vi "Command - Continuous (SubVI) - A.vi"(0 "ESP Config":T1={"COM Port Input"="COM8", "Manual Command"={"Device Type"="", "Instance"="", "Command"="", "Sub-Command"="", "Parameters (Seperate by :)"=""}, "Device Type"="e", "Instance"="a", "Use Manual Command"=FALSE, "Timeout [msec]"=1000, "Read/Write Wait [msec]"=50}, 5 "ESP Table Cluster Ref":refnum<vi>, 7 "Display Cluster Ref":refnum<vi>) -> (4 "ESP Values":T2, 6 "Parameters":string[][](array[string]), 8 "Continuous Header":string[](array[string]), 10 "Continuous Data":string[](array[string]), 15 "CONTINUOUS ERR":errorcluster)   [LabVIEW 2011]
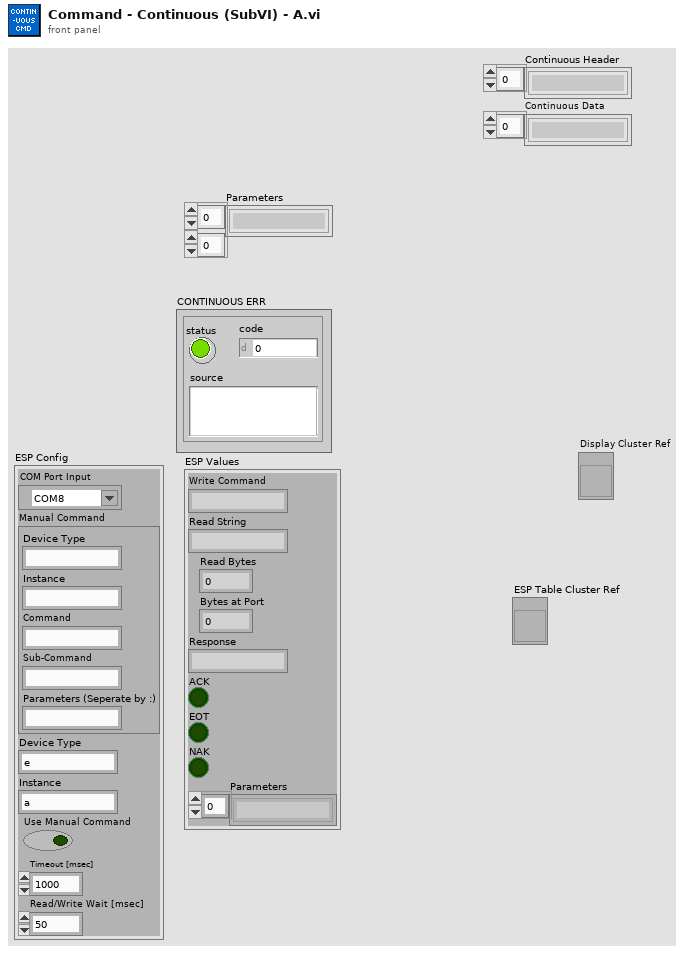
[diagram p1: front panel]
types:
  T1 = cluster{"COM Port Input":refnum<visa-resource-name>, "Manual Command":cluster{"Device Type":string, "Instance":string, "Command":string, "Sub-Command":string, "Parameters (Seperate by :)":string}, "Device Type":string, "Instance":string, "Use Manual Command":bool, "Timeout [msec]":u32, "Read/Write Wait [msec]":u32}
  T2 = cluster{"Write Command":string, "Read String":string, "Read Bytes":u32, "Bytes at Port":u32, "Response":string, "ACK":bool, "EOT":bool, "NAK":bool, "Parameters":string[]}
  T3 = cluster{"ON Demand Button":i32, "ON Demand Commands":i32, "Continuous Button":i32, "Continuous Commands":i32, "Error Button":i32, "Error Command":i32, "Status Button":i32, "Status Command":i32, "Digital Button":i32, "Digital Command":i32, "Save Table Button":i32, "Active Table":i32, "New Table Name":i32, "Table":i32}
  T4 = cluster{"Device Type":string, "Instance":string, "Command":string, "Sub-Command":string, "Parameters (Seperate by :)":string}
  T5 = cluster{"CMD_Display":string, "Param Output":string[][]}[]
  T6 = cluster{"ParamName":string, "Param Output":string[][]}
  T7 = cluster{"ParamName":string, "Param Output":string[][]}[]
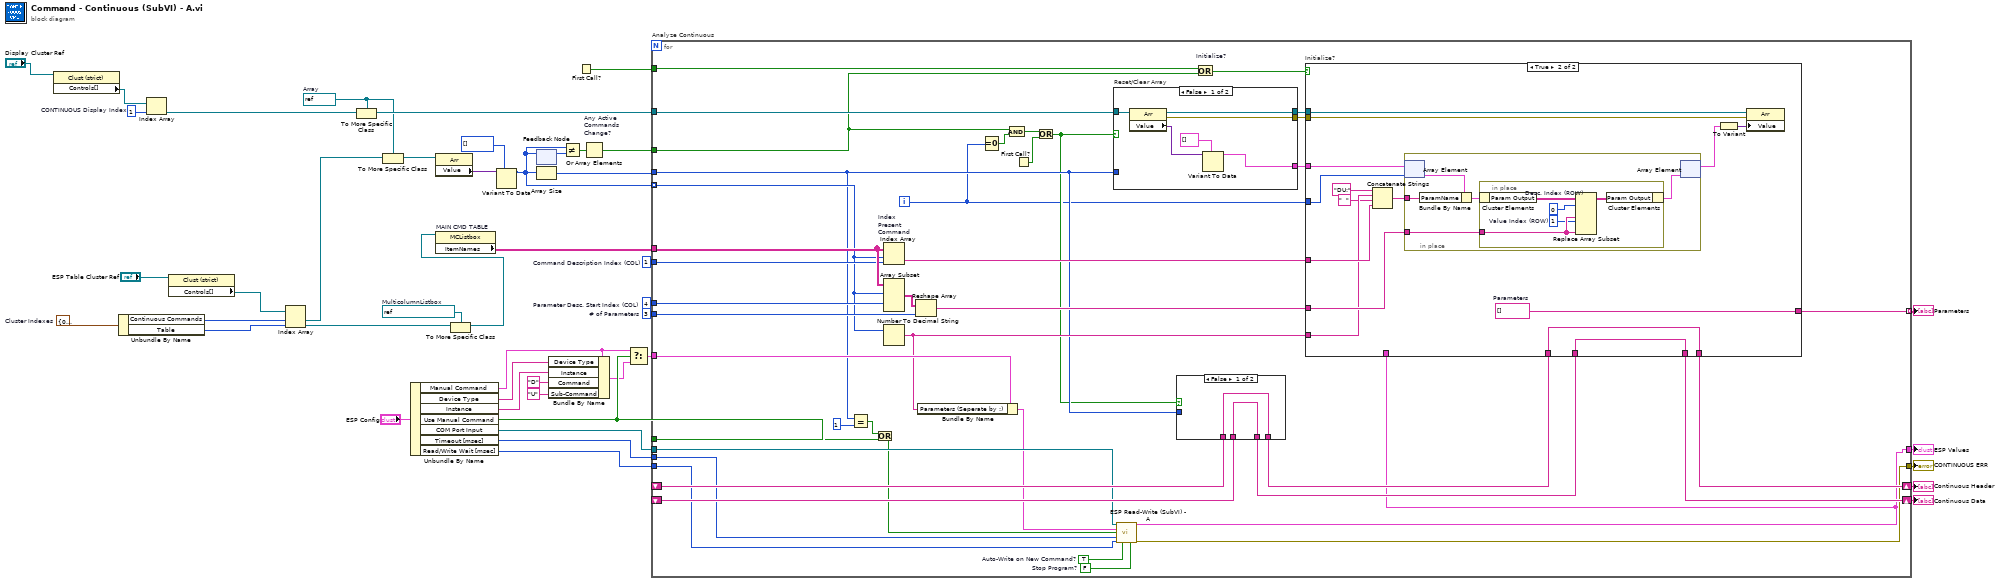
[diagram p0: block diagram]
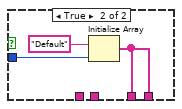
[diagram p2: hidden frame]
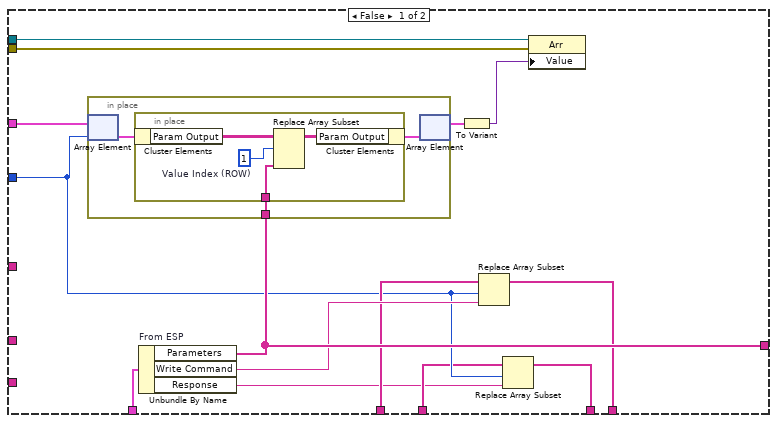
[diagram p3: hidden frame]
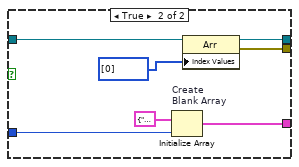
[diagram p4: hidden frame]
diagram:
  w9 = 1  # CONTINUOUS Display Index
  w12 = refnum<vi> refnum  # MulticolumnListbox
  w17 = T3 {"ON Demand Button"=0, "ON Demand Commands"=1, "Continuous Button"=2, "Continuous Commands"=3, "Error Button"=4, "Error Command"=5, "Status Button"=6, "Status Command"=7, "Digital Button"=8, "Digital Command"=9, "Save Table Button"=10, "Active Table"=11, "New Table Name"=12, "Table"=13}  # Cluster Indexes
  w4 = refnum<vi> refnum  # Array
  w43 = 1  # Command Description Index (COL)
  w44 = 3  # # of Parameters
  w45 = 4  # Parameter Desc. Start Index (COL)
  n1 = property class="Clust (strict)"(reference="Display Cluster Ref") -> ("Controls[]"=w10:refnum<vi>[])  [unwired: 1 in, 2 out]
  n2 = Unbundle By Name(w17) -> ("Continuous Commands"=w16:i32, "Table"=w15:i32)
  n3 = Index Array(array=w10, index=w9) -> (element=w8:refnum<vi>)
  n4 = property class="Clust (strict)"(reference="ESP Table Cluster Ref") -> ("Controls[]"=w18:refnum<vi>[])  [unwired: 1 in, 2 out]
  n5 = Index Array(array=w18, index #1=w16, index #2=w15) -> (element #1=w2:refnum<vi>, element #2=w13:refnum<vi>)
  n6 = To More Specific Class(target class=w4, reference=w8) -> (specific class reference=w19:refnum<vi>)  [unwired: 1 in, 1 out]
  n7 = To More Specific Class(target class=w4, reference=w2) -> (specific class reference=w5:refnum<vi>)  [unwired: 1 in, 1 out]
  n8 = Unbundle By Name("ESP Config") -> ("Manual Command"=w32:T4, "Device Type"=w34:string, "Instance"=w33:string, "Use Manual Command"=w39:bool, "COM Port Input"=w40:refnum<visa-resource-name>, "Timeout [msec]"=w41:u32, "Read/Write Wait [msec]"=w42:u32)
  n9 = property class="Arr"(reference=w5) -> ("Value"=w6:variant)  [unwired: 1 in, 2 out]
  n10 = To More Specific Class(target class=w12, reference=w13) -> (specific class reference=w11:refnum<vi>)  [unwired: 1 in, 1 out]
  n11 = property on="MAIN CMD TABLE" class="MCListbox"(reference=w11) -> ("ItemNames"=w25:string[][])  [unwired: 1 in, 2 out]
  n12 = Variant To Data(type=i32[] [], Variant=w6) -> (data=w3:i32[])  [unwired: 1 in, 1 out]
  n13 = feedback #1() -> (w27:i32[])  [unwired: 1 in]
  n14 = feedback-in #1(w3) -> ()
  n15 = Array Size(array=w3) -> (size(s)=w28:i32)
  n16 = Bundle By Name(cluster=w32, "Device Type"=w34, "Instance"=w33, "Command"="D", "Sub-Command"="U") -> (w31:T4)
  n17 = Not Equal?(x=w3, y=w27) -> (x != y?=w26:bool[])
  n18 = First Call?() -> (First Call?: T/F=w30:bool)
  n19 = Or Array Elements "Any Active\nCommands\nChange?"(Boolean array=w26) -> (logical OR=w29:bool)
  n20 = Select(t=w32, s=w39, f=w31) -> (s? t:f=w37:T4)
  n21 = for "Analyze Continuous" {
    tunnel: w25 -> [w86]
    tunnel: w30 -> [w80]
    tunnel: w19 -> [w79]
    tunnel: w28 -> [w64]
    tunnel: w45 -> [w83]
    tunnel: w37 -> [w87]
    tunnel: [w47] -> w23
    tunnel: w41 -> [w52]
    tunnel: w44 -> [w82]
    tunnel: w29 -> [w74]
    tunnel: w39 -> [w53]
    tunnel: w40 -> [w55]
    tunnel: w42 -> [w51]
    tunnel: w3 -> [w67] mode=indexing
    tunnel: w43 -> [w68]
    tunnel: [w65] -> w22 mode=indexing
    tunnel: [w48] -> w24
    shift-right: [w56] -> w21
    shift-left: _ -> [w62]
    shift-right: [w57] -> w20
    shift-left: _ -> [w61]
    i -> [w60]
    w49 = FALSE  # Stop Program?
    w50 = TRUE  # Auto-Write on New Command?
    n22 = Equal?(x=w64, y=1) -> (x = y?=w72:bool)
    n23 = Or(x=w72, y=w53) -> (x .or. y?=w46:bool)
    n24 = Index Array "Index\nPresent\nCommand"(array=w86, index (row)=w67, index (col)=w68) -> (element=w66:string)
    n25 = Array Subset(array=w86, index (row)=w67, index (col)=w83) -> (w85:string[][])  [unwired: 2 in]
    n26 = Number To Decimal String(number=w67) -> (decimal integer string=w81:string)  [unwired: 1 in]
    n27 = Reshape Array(w85, w82) -> (w84:string[])
    n28 = Bundle By Name(cluster=w87, "Parameters (Seperate by :)"=w81) -> (w54:T4)
    n29 = Equal To 0?(x=w60) -> (x = 0?=w78:bool)
    n30 = And(x=w74, y=w78) -> (x .and. y?=w71:bool)
    n31 = First Call?() -> (First Call?: T/F=w70:bool)
    n32 = Or(x=w71, y=w70) -> (x .or. y?=w63:bool)
    n33 = case "Reset/Clear Array" shown="False" w63 {
      tunnel: w79 -> [w144 w149]
      tunnel: [w143 w147] -> w75
      tunnel: [w142 w148] -> w76
      tunnel: [w139 w150] -> w77
      tunnel: w64 -> [_ w151]
      frame False {
        n34 = property class="Arr"(reference=w144) -> (reference out=w142:refnum<vi>, error out=w143:errorcluster, "Value"=w141:variant)  [unwired: 1 in]
        n35 = Variant To Data(type=T5 [], Variant=w141) -> (data=w139:T5)  [unwired: 1 in, 1 out]
      }
      frame True {
        n36 = Initialize Array "Create\nBlank Array"(T6 {"ParamName"="", "Param Output"=[["", "", ""], [" ", "", ""]]} ("Read Value\nCluster"), w151) -> (w150:T7)
        n37 = property class="Arr"(reference=w149, "Index Values"=u32[] [0]) -> (reference out=w148:refnum<vi>, error out=w147:errorcluster)  [unwired: 1 in]
      }
    }
    n38 = call "ESP Read-Write (SubVI) - A.vi"("COM Port Input"=w55, "Command Input"=w54, "Manual Write Command"=w46, "Timeout (ms)"=w52, "Write/Read Wait (ms)"=w51, "Auto-Write on New Command?"=w50, "Stop Program?"=w49) -> ("ESP Values"=w47:T2, "Error Output"=w48:errorcluster)  [unwired: 7 in]
    n39 = case shown="False" w63 {
      tunnel: w64 -> [_ w92]
      tunnel: [w88 w90] -> w58
      tunnel: [w89 w90] -> w59
      tunnel: w62 -> [w89 _]
      tunnel: w61 -> [w88 _]
      frame False {
      }
      frame True {
        n40 = Initialize Array("Default", w92) -> (w90:string[])
      }
    }
    n41 = Or "Initialize?"(x=w80, y=w74) -> (x .or. y?=w69:bool)
    n42 = case "Initialize?" shown="True" w69 {
      tunnel: w66 -> [_ w128]
      tunnel: w84 -> [_ w127]
      tunnel: w60 -> [w97 w126]
      tunnel: w81 -> [_ w125]
      tunnel: w77 -> [w106 w124]
      tunnel: w76 -> [w105 w123]
      tunnel: w75 -> [w104 w122]
      tunnel: w47 -> [w102 _]
      tunnel: [w101 w117] -> w65
      tunnel: w59 -> [w98 w116]
      tunnel: w58 -> [w95 w115]
      tunnel: [w99 w116] -> w56
      tunnel: [w96 w115] -> w57
      frame False {
        n43 = Unbundle By Name "From ESP"(w102) -> ("Parameters"=w101:string[], "Write Command"=w100:string, "Response"=w94:string)
        n44 = in-place {
          in-place-border: w101 -> [w107]
          n45 = in-place-array #2(w106, w97) -> (w108:T6)
          n46 = in-place {
            in-place-border: w107 -> [w110]
            w112 = 1  # Value Index (ROW)
            n47 = in-place-cluster #3(w108) -> ("Param Output"=w113:string[][])
            n48 = Replace Array Subset(array=w113, new element=w110, index (row)=w112) -> (w111:string[][])  [unwired: 1 in]
            n49 = in-place-cluster #3("Param Output"=w111) -> (w109:T6)
          }
          n50 = in-place-array #2(w109) -> (w103:T7)  [unwired: 1 out]
        }
        n51 = To Variant(anything=w103) -> (Variant=w93:variant)
        n52 = Replace Array Subset(array=w98, new element=w100, index=w97) -> (w99:string[])
        n53 = Replace Array Subset(array=w95, new element=w94, index=w97) -> (w96:string[])
        n54 = property class="Arr"(reference=w105, error in=w104, "Value"=w93) -> ()  [unwired: 2 out]
      }
      frame True {
        w117 = string[] []  # Parameters
        n55 = Concatenate Strings("DU:" ("string"), w125, "  ", w128) -> (w120:string)
        n56 = in-place {
          in-place-border: w120 -> [w130]
          in-place-border: w127 -> [w129]
          n57 = in-place-array #4(w124, w126) -> (w133:T6)
          n58 = Bundle By Name(cluster=w133, "ParamName"=w130) -> (w132:T6)
          n59 = in-place {
            in-place-border: w129 -> [w137]
            w135 = 1  # Value Index (ROW)
            w136 = 0  # Desc. Index (ROW)
            n60 = in-place-cluster #5(w132) -> ("Param Output"=w134:string[][])
            n61 = Replace Array Subset(array=w134, new element #1=w137, index (row) #1=w136, new element #2=w137, index (row) #2=w135) -> (w138:string[][])  [unwired: 2 in]
            n62 = in-place-cluster #5("Param Output"=w138) -> (w131:T6)
          }
          n63 = in-place-array #4(w131) -> (w121:T7)  [unwired: 1 out]
        }
        n64 = To Variant(anything=w121) -> (Variant=w114:variant)
        n65 = property class="Arr"(reference=w123, error in=w122, "Value"=w114) -> ()  [unwired: 2 out]
      }
    }
  }
  "CONTINUOUS ERR" <- w24
  "ESP Values" <- w23
  "Parameters" <- w22
  "Continuous Header" <- w21
  "Continuous Data" <- w20
